vi "Tx Queue Status to DBLs.vi"(3 "TxQueueStatus":T1 {"QueueStatus" items=["FDX_QUE_EMPTY", "FDX_QUE_FILLED", "FDX_QUE_FULL", "FDX_QUE_SENT", "FDX_QUE_CYCL_RUN", "FDX_QUE_CYCL_SENT"]}) -> (1 "TxQueueStatusDBLs":dbl[](array[numeric]))   [LabVIEW 2020, in "AIM ARINC 664 Engine.lvlib" / "Implementation.lvlib" / "Tx Generic Execution Unit.lvclass"]
uses:
  Tx Generic Execution Unit.lvclass
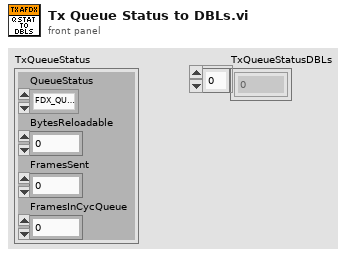
[diagram p1: front panel]
types:
  T1 = cluster{"QueueStatus":i32, "BytesReloadable":u32, "FramesSent":u32, "FramesInCycQueue":u32}
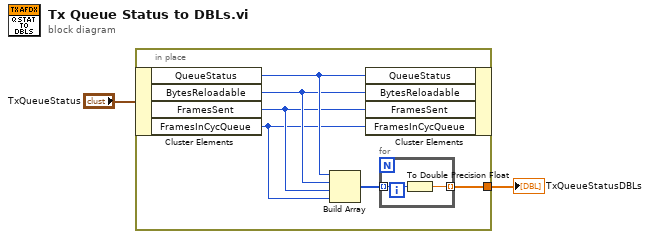
[diagram p0: block diagram]
diagram:
  n1 = in-place {
    in-place-border: [w3] -> w1
    n2 = in-place-cluster #1("TxQueueStatus") -> ("QueueStatus"=w8:i32, "BytesReloadable"=w7:u32, "FramesSent"=w6:u32, "FramesInCycQueue"=w5:u32)
    n3 = Build Array(w8, w7, w6, w5) -> (w4:u32[])
    n4 = in-place-cluster #1("QueueStatus"=w8, "BytesReloadable"=w7, "FramesSent"=w6, "FramesInCycQueue"=w5) -> ()  [unwired: 1 out]
    n5 = for {
      tunnel: w4 -> [w10] mode=indexing
      tunnel: [w9] -> w3 mode=indexing
      n6 = To Double Precision Float(number=w10) -> (double precision float=w9:dbl)
    }
  }
  "TxQueueStatusDBLs" <- w1
